vi "SPD.DT Meas DT_Grid.vi"(5 "Continue":refnum<vi>, 7 "Progress":refnum<vi>, 8 "Error In":errorcluster, 11 "SPD.Stand Ctrl in":T2={"spdDeviceSession"={"spdRef"=0, "connected"=FALSE, "spdName"="", "specification"={"diod case"=enum."default", "type"=enum."Unknown", "frequency"=enum."Unknown"}, "hidSPD.Controller"={"TSet"=0.0, "HV_bias"=0.0, "DDS_stb_code"=0}, "hidSPD.Sturtup Values"={"TSet"=0.0, "HV_bias"=0.0, "DDS_stb_code"=0}}, "DevBSession"={"DevBRef"="", "connected"=FALSE}, "FreqCSession"={"FreqCRef"="", "timeout"=0.0, "Gate"=0.0, "connected"=FALSE}, "8164BSession"={"Connection ID"=refnum, "Connected"=FALSE, "Info"="", "Slots Info"=[]}, "LeCroySession"={"LeCroySession"="", "connected"=FALSE}, "Events"={"DCRTest"=refnum, "Stop"=refnum}, "configFile"={"configFile ref"=refnum, "configFile path"=path "", "equipmentFile ref"=refnum}, "SPD.Meas Grid"={"DateTime"="", "DT"=[], "Insensitivity"=[], "Temprature"=[], "Stb_code"=[], "HV_Bias"=[]}, "SPD.Queues"={"state queue"=refnum}, "Console"=refnum} {"spdDeviceSession"."hidSPD.Sturtup Values"."HV_bias" format="%#_6p, V"; "spdDeviceSession"."hidSPD.Sturtup Values"."TSet" format="%#_6p, DegC"; "spdDeviceSession"."hidSPD.Controller"."HV_bias" format="%#_6p, V"; "spdDeviceSession"."hidSPD.Controller"."TSet" format="%#_6p, DegC"}) -> (0 "Error Out":errorcluster, 1 "pass":bool, 2 "Report":string, 3 "SPD.Stand Ctrl out":T2={"spdDeviceSession"={"spdRef"=0, "connected"=FALSE, "spdName"="", "specification"={"diod case"=enum."default", "type"=enum."Unknown", "frequency"=enum."Unknown"}, "hidSPD.Controller"={"TSet"=0.0, "HV_bias"=0.0, "DDS_stb_code"=0}, "hidSPD.Sturtup Values"={"TSet"=0.0, "HV_bias"=0.0, "DDS_stb_code"=0}}, "DevBSession"={"DevBRef"="", "connected"=FALSE}, "FreqCSession"={"FreqCRef"="", "timeout"=0.0, "Gate"=0.0, "connected"=FALSE}, "8164BSession"={"Connection ID"=refnum, "Connected"=FALSE, "Info"="", "Slots Info"=[]}, "LeCroySession"={"LeCroySession"="", "connected"=FALSE}, "Events"={"DCRTest"=refnum, "Stop"=refnum}, "configFile"={"configFile ref"=refnum, "configFile path"=path "", "equipmentFile ref"=refnum}, "SPD.Meas Grid"={"DateTime"="", "DT"=[], "Insensitivity"=[], "Temprature"=[], "Stb_code"=[], "HV_Bias"=[]}, "SPD.Queues"={"state queue"=refnum}, "Console"=refnum} {"spdDeviceSession"."hidSPD.Sturtup Values"."HV_bias" format="%#_6p, V"; "spdDeviceSession"."hidSPD.Sturtup Values"."TSet" format="%#_6p, DegC"; "spdDeviceSession"."hidSPD.Controller"."HV_bias" format="%#_6p, V"; "spdDeviceSession"."hidSPD.Controller"."TSet" format="%#_6p, DegC"})   [LabVIEW 2018]
uses:
  typedefs/SPD.Stand Ctrl.ctl
  Instruments/SPD HID Interface/hidSPDLibForLabView/LibVIs/hidSPD Controls/hidSPD Device Session.ctl
  Instruments/SPD HID Interface/hidSPDLibForLabView/LibVIs/hidSPD Controls/hidSPD.SPD specification.ctl
  Instruments/SPD HID Interface/hidSPDLibForLabView/LibVIs/hidSPD Controls/hidSPD SPD Diod Case.ctl
  Instruments/SPD HID Interface/hidSPDLibForLabView/LibVIs/hidSPD Controls/hidSPD SPD Type.ctl
  Instruments/SPD HID Interface/hidSPDLibForLabView/LibVIs/hidSPD Controls/hidSPD.STB Frequency.ctl
  Instruments/SPD HID Interface/hidSPDLibForLabView/LibVIs/hidSPD Controls/hidSPD Controller.ctl
  Instruments/KC705 DevBoard/typedefs/DevB.Session.ctl
  Instruments/KeySight 53230A/typedefs/FreqC.Session.ctl
  Instruments/KeySight 8164B/KeySight 8164B LAN InstrLib/typedefs/KeySight 8164B control.ctl
  Instruments/LeCroy SDA830/typedefs/LeCroy.Session.ctl
  typedefs/SPD.Events.ctl
  ConfigFile/SPD.Config File ctrl.ctl
  <vilib>/Utility/config.llb/Config Data RefNum.ctl
  typedefs/SPD.Meas Grid.ctl
  typedefs/SPD.Queues.ctl
  typedefs/SPD.Stand state.ctl
  typedefs/SPD.Common HW Setup ctr.ctl
  typedefs/SPD.QE Strobe_Phase Tune Limits.ctl
  <vilib>/Analysis/1siggen.llb/Ramp Pattern by Delta.vi
  <vilib>/Analysis/NI_AALBase.lvlib
  Instruments/KeySight 8164B/KeySight 8164B LAN InstrLib.lvlib
  <vilib>/Utility/config.llb/NI_LVConfig.lvlib
  Instruments/SPD HID Interface/hidSPDLibForLabView/hidSPDLibForLabView.lvlib
panel:
  out "XY Graph":T1(graph)
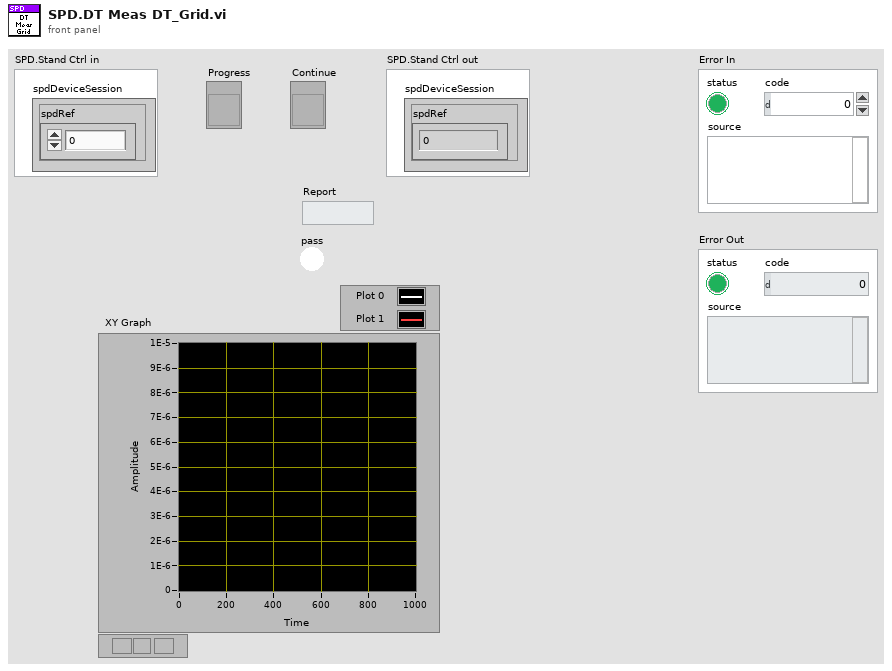
[diagram p1: front panel]
types:
  T1 = cluster{"result out":dbl[], "result out":dbl[]}[]
  T2 = typedef "SPD.Stand Ctrl.ctl" = cluster{"spdDeviceSession":T3, "DevBSession":T9, "FreqCSession":T10, "8164BSession":T11, "LeCroySession":T12, "Events":T13, "configFile":T14, "SPD.Meas Grid":T16, "SPD.Queues":T17, "Console":refnum<vi>}
  T3 = typedef "hidSPDLibForLabView.lvlib/hidSPD Device Session.ctl" = cluster{"spdRef":u64, "connected":bool, "spdName":string, "specification":T4, "hidSPD.Controller":T8, "hidSPD.Sturtup Values":T8}
  T4 = typedef "hidSPDLibForLabView.lvlib/hidSPD.SPD specification.ctl" = cluster{"diod case":T5, "type":T6, "frequency":T7}
  T5 = typedef "hidSPDLibForLabView.lvlib/hidSPD SPD Diod Case.ctl" = enum16{"Unknown", "default", "butterfly"}
  T6 = typedef "hidSPDLibForLabView.lvlib/hidSPD SPD Type.ctl" = enum16{"Unknown", "Free Run", "Gate"}
  T7 = typedef "hidSPDLibForLabView.lvlib/hidSPD.STB Frequency.ctl" = enum16{"Unknown", "312", "1250"}
  T8 = typedef "hidSPDLibForLabView.lvlib/hidSPD Controller.ctl" = cluster{"TSet":sgl, "HV_bias":sgl, "DDS_stb_code":u16}
  T9 = typedef "DevB.Session.ctl" = cluster{"DevBRef":refnum<visa-resource-name>, "connected":bool}
  T10 = typedef "FreqC.Session.ctl" = cluster{"FreqCRef":refnum<visa-resource-name>, "timeout":dbl, "Gate":dbl, "connected":bool}
  T11 = typedef "KeySight 8164B LAN InstrLib.lvlib/KeySight 8164B control.ctl" = cluster{"Connection ID":refnum<k5>, "Connected":bool, "Info":string, "Slots Info":string[]}
  T12 = typedef "LeCroy.Session.ctl" = cluster{"LeCroySession":refnum<visa-resource-name>, "connected":bool}
  T13 = typedef "SPD.Events.ctl" = cluster{"DCRTest":refnum<user-event>, "Stop":refnum<user-event>}
  T14 = typedef "SPD.Config File ctrl.ctl" = cluster{"configFile ref":T15, "configFile path":path, "equipmentFile ref":T15}
  T15 = typedef "NI_LVConfig.lvlib/Config Data RefNum.ctl" = refnum<k1>
  T16 = typedef "SPD.Meas Grid.ctl" = cluster{"DateTime":string, "DT":dbl[], "Insensitivity":dbl[], "Temprature":dbl[], "Stb_code":dbl[], "HV_Bias":dbl[][][][]}
  T17 = typedef "SPD.Queues.ctl" = cluster{"state queue":refnum<queue>}
  T18 = typedef "SPD.Common HW Setup ctr.ctl" = cluster{"FS":i32, "TS":i32, "Gate":dbl, "Att1 enable":bool, "Att3 enable":bool, "Att3 Att":dbl, "Scope setup file path":string, "Pset":dbl, "Set Pset":bool}
  T19 = typedef "SPD.DT&Insens Test Params.ctl" = cluster{"FS":i32, "TS":i32, "Att3":dbl, "Gate":dbl, "Num of Meas":i32, "ScopeRecallFile":string, "HistoSize":i32, "DT_min":u16, "DT_max":u16, "DT_step":u16, "Desired_DTs":dbl[], "Insens_bound":u16, "Insens_step":u16}
  T20 = typedef "SPD.QE Strobe_Phase Tune Limits.ctl" = cluster{"ph_start":i32, "ph_stop":i32, "ph_step":i32}
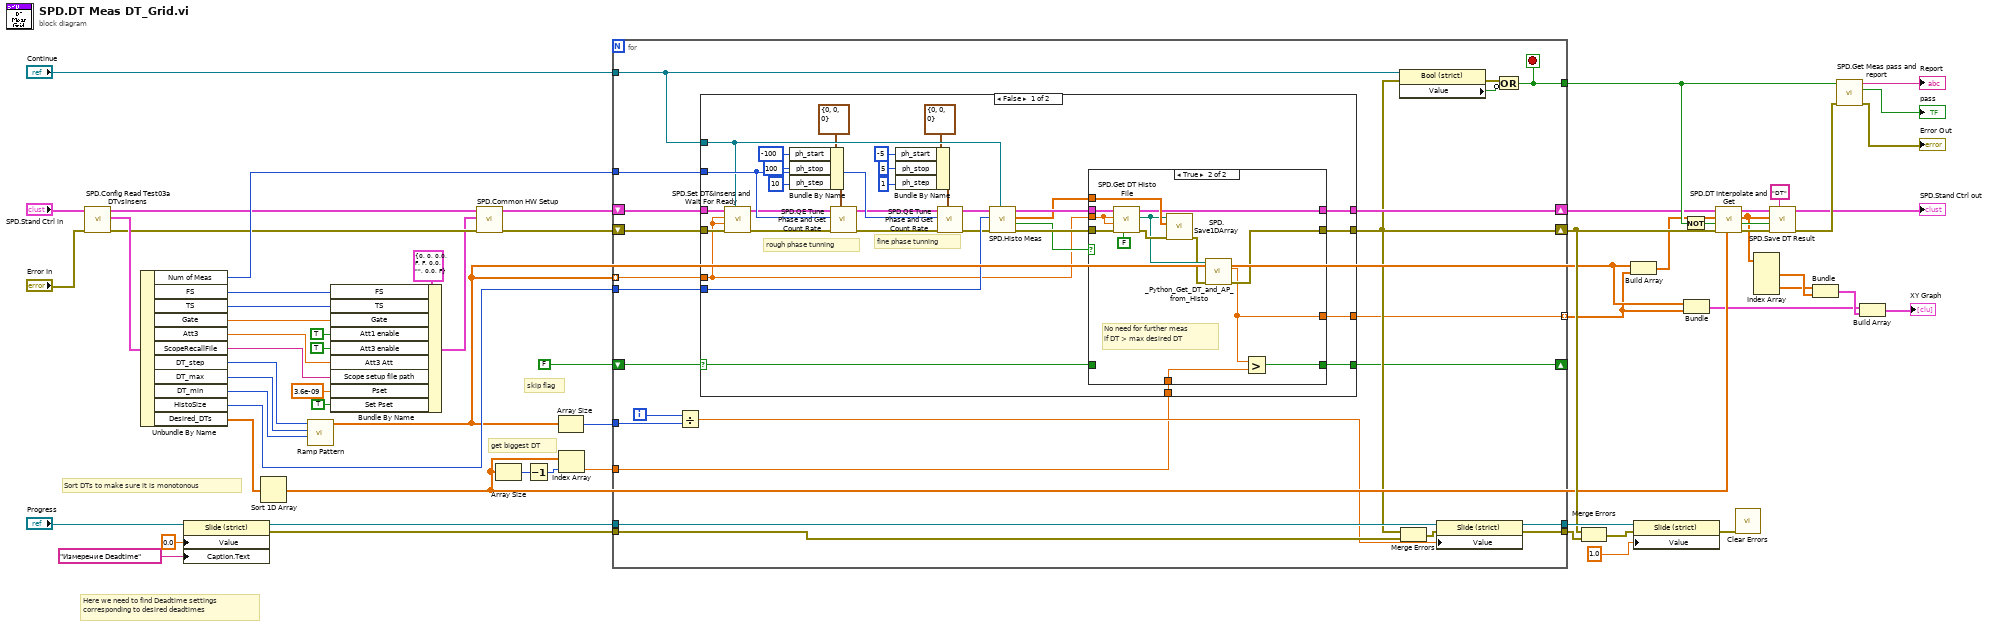
[diagram p0: block diagram]
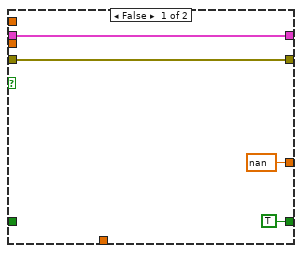
[diagram p2: hidden frame]
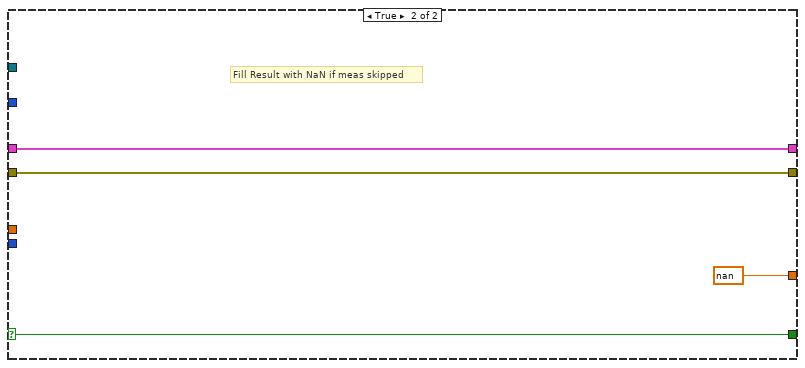
[diagram p3: hidden frame]
diagram:
  # "get biggest DT"
  # "Sort DTs to make sure it is monotonous"
  # "skip flag"
  # "Here we need to find Deadtime settings \ncorresponding to desired deadtimes"
  n1 = call "SPD.Config Read Test03a DTvsInsens.vi"("Error In"="Error In", "SPD.Stand Ctrl in"="SPD.Stand Ctrl in") -> ("Error Out"=w40:errorcluster, "DTvsInsens Params"=w41:T19, "SPD.Stand Ctrl out"=w43:T2)  [unwired: 7 in]
  n2 = Unbundle By Name(w41) -> ("Num of Meas"=w59:i32, "FS"=w48:i32, "TS"=w47:i32, "Gate"=w38:dbl, "Att3"=w37:dbl, "ScopeRecallFile"=w36:string, "DT_step"=w33:u16, "DT_max"=w32:u16, "DT_min"=w31:u16, "HistoSize"=w29:i32, "Desired_DTs"=w14:dbl[])
  n3 = property class="Slide (strict)"(reference="Progress", "Value"=0.0, "Caption.Text"="Измерение Deadtime") -> (reference out=w55:refnum<vi>, error out=w53:errorcluster)  [unwired: 1 in]
  n4 = Sort 1D Array(array=w14) -> (sorted array=w10:dbl[])
  n5 = call-poly <vilib>:"Ramp Pattern.vi"("start"=w31, "end"=w32, "delta"=w33) -> ("Ramp Pattern"=w8:dbl[])  [unwired: 6 in, 2 out]
  n6 = Bundle By Name(cluster=T18 {"FS"=0, "TS"=0, "Gate"=0.0, "Att1 enable"=FALSE, "Att3 enable"=FALSE, "Att3 Att"=0.0, "Scope setup file path"="", "Pset"=0.0, "Set Pset"=FALSE} ("common hw setup"), "FS"=w48, "TS"=w47, "Gate"=w38, "Att1 enable"=TRUE, "Att3 enable"=TRUE, "Att3 Att"=w37, "Scope setup file path"=w36, "Pset"=3.6e-09, "Set Pset"=TRUE) -> (w39:T18)
  n7 = call "SPD.Common HW Setup.vi"("error in (no error)"=w40, "common hw setup"=w39, "SPD.Stand Ctrl in in"=w43) -> ("error out"=w24:errorcluster, "SPD.Stand Ctrl out"=w23:T2)  [unwired: 7 in]
  n8 = Array Size(array=w10) -> (size(s)=w13:i32)
  n9 = Decrement(x=w13) -> (x-1=w12:i32)
  n10 = Array Size(array=w8) -> (size(s)=w30:i32)
  n11 = Index Array(array=w10, index=w12) -> (element=w11:dbl)
  n12 = for {
    shift-right: [w86] -> w26
    shift-left: w23 -> [w79]
    shift-right: [w70] -> w25
    shift-left: w24 -> [w78]
    tunnel: "Continue" -> [w77]
    tunnel: [w85] -> w28
    tunnel: w55 -> [w84]
    tunnel: [w83] -> w62
    tunnel: w59 -> [w82]
    tunnel: w53 -> [w81]
    tunnel: [w80] -> w51
    tunnel: w8 -> [w69] mode=indexing
    tunnel: w30 -> [w68]
    tunnel: w29 -> [w71]
    shift-right: [w66] -> _
    shift-left: FALSE -> [w67]
    tunnel: w11 -> [w65]
    tunnel: [w64] -> w7 mode=indexing
    i -> [w72]
    stop <- w85 stop-if-true
    n13 = Divide(x=w72, y=w68) -> (x/y=w74:dbl)
    n14 = case shown="False" w67 {
      selector: w67 -> [w90 w137]
      tunnel: [w118 w139] -> w86
      tunnel: w82 -> [w117 _]
      tunnel: w79 -> [w116 w139]
      tunnel: w78 -> [w114 w138]
      tunnel: w77 -> [w113 _]
      tunnel: w71 -> [w111 _]
      tunnel: [w92 w138] -> w70
      tunnel: w69 -> [w91 _]
      tunnel: [w87 nan] -> w64
      tunnel: [w89 w137] -> w66
      tunnel: w65 -> [w88 _]
      frame False {
        # "fine phase tunning"
        # "rough phase tunning"
        n15 = call "SPD.Set DT&Insens and Wait For Ready.vi"("Continue"=w113, "Error In"=w114, "insensitivity"=w91, "deadtime"=w91, "SPD.Stand Ctrl in"=w116) -> ("Error Out"=w112:errorcluster, "SPD.Stand Ctrl out"=w115:T2)  [unwired: 5 in]
        n16 = Bundle By Name(cluster=T20 {"ph_start"=0, "ph_stop"=0, "ph_step"=0} ("SPD.QE Strobe_Phase Tune Limits"), "ph_start"=-100, "ph_stop"=100, "ph_step"=10) -> (w95:T20)
        n17 = call "SPD.QE Tune Phase and Get Count Rate.vi"("SPD.QE Strobe_Phase Tune Limits"=w95, "Error In"=w112, "Num of FreqC Meas"=w117, "SPD.Stand Ctrl in"=w115) -> ("Error Out"=w100:errorcluster, "SPD.Stand Ctrl out"=w101:T2)  [unwired: 4 in, 2 out]
        n18 = Bundle By Name(cluster=T20 {"ph_start"=0, "ph_stop"=0, "ph_step"=0} ("SPD.QE Strobe_Phase Tune Limits"), "ph_start"=-5, "ph_stop"=5, "ph_step"=1) -> (w105:T20)
        n19 = call "SPD.QE Tune Phase and Get Count Rate.vi"("SPD.QE Strobe_Phase Tune Limits"=w105, "Error In"=w100, "Num of FreqC Meas"=w117, "SPD.Stand Ctrl in"=w101) -> ("Error Out"=w93:errorcluster, "SPD.Stand Ctrl out"=w94:T2)  [unwired: 4 in, 2 out]
        n20 = call "SPD.Histo Meas.vi"("Continue"=w113, "Error In"=w93, "Histo length"=w111, "SPD.Stand Ctrl in"=w94) -> ("Error Out"=w108:errorcluster, "pass"=w107:bool, "Histo"=w109:dbl[], "SPD.Stand Ctrl out"=w110:T2)  [unwired: 4 in]
        n21 = case shown="True" w107 {
          tunnel: [w122 w130] -> w118
          tunnel: [w121 w127] -> w92
          tunnel: w110 -> [w122 w135]
          tunnel: w109 -> [_ w132]
          tunnel: w108 -> [w121 w133]
          tunnel: w91 -> [_ w134]
          tunnel: [nan ("Dead Time") w123] -> w87
          tunnel: w90 -> [_ _]
          tunnel: [TRUE w126] -> w89
          tunnel: w88 -> [_ w124]
          frame False {
          }
          frame True {
            # "No need for further meas \nif DT > max desired DT"
            n22 = call "SPD.Get DT Histo File.vi"("DT folder"=FALSE, "Error In"=w133, "DT"=w134, "Insens"=w134, "SPD.Stand Ctrl in"=w135) -> ("Error Out"=w131:errorcluster, "DT Results path"=w129:path, "SPD.Stand Ctrl out"=w130:T2)  [unwired: 4 in]
            n23 = call "SPD.Save1DArray.vi"("Error In"=w131, "Array"=w132, "File Path"=w129) -> ("Error Out"=w128:errorcluster)  [unwired: 8 in]
            n24 = call "_Python_Get_DT_and_AP_from_Histo.vi"("error in (no error)"=w128, "Histo path"=w129) -> ("error out"=w127:errorcluster, "Dead Time"=w123:dbl)  [unwired: 7 in, 1 out]
            n25 = Greater?(x=w123, y=w124) -> (0:w126:bool)
          }
        }
      }
      frame True {
        # "Fill Result with NaN if meas skipped"
      }
    }
    n26 = property class="Bool (strict)"(reference=w77, error in=w70) -> (error out=w75:errorcluster, "Value"=w76:bool)  [unwired: 1 out]
    n27 = Merge Errors(w70, w81) -> (w73:errorcluster)
    n28 = property class="Slide (strict)"(reference=w84, error in=w73, "Value"=w74) -> (reference out=w83:refnum<vi>, error out=w80:errorcluster)
    n29 = Compound Arithmetic op=OR(w75, invert w76) -> (w85:bool)
  }
  n30 = Merge Errors(w25, w51) -> (w52:errorcluster)
  n31 = Build Array(w8, w7) -> (w9:dbl[][])
  n32 = property class="Slide (strict)"(reference=w62, error in=w52, "Value"=1.0) -> (error out=w60:errorcluster)  [unwired: 1 out]
  n33 = Not(x=w28) -> (.not. x?=w18:bool)
  n34 = Bundle("Ramp Pattern"=w8, w7) -> (w4:cluster{"Ramp Pattern":dbl[], dbl[]})  [unwired: 1 in]
  n35 = call "SPD.DT Interpolate and Get.vi"("desired DT"=w10, "Error In"=w25, "valid in"=w18, "Result"=w9, "SPD.Stand Ctrl in"=w26) -> ("Error Out"=w19:errorcluster, "valid out"=w17:bool, "result out"=w6:dbl[][], "SPD.Stand Ctrl out"=w20:T2)  [unwired: 3 in]
  n36 = call <vilib>:"Clear Errors.vi"("error in (no error)"=w60) -> ()  [unwired: 5 in, 2 out]
  n37 = Index Array(array=w6) -> (element #1=w2:dbl[], element #2=w1:dbl[])  [unwired: 4 in]
  n38 = call "SPD.Save DT Result.vi"("Name"="DT", "Error In"=w19, "write to file"=w17, "Result"=w6, "SPD.Stand Ctrl in"=w20) -> ("Error Out"=w16:errorcluster, "SPD.Stand Ctrl out"=→"SPD.Stand Ctrl out":T2)  [unwired: 5 in]
  n39 = Bundle("result out"=w1, "result out"=w2) -> (w5:cluster{"result out":dbl[], "result out":dbl[]})  [unwired: 1 in]
  n40 = call "SPD.Get Meas pass and report.vi"("error in (no error)"=w16, "error or stoped"=w28) -> ("error out"=→"Error Out":errorcluster, "pass"=→"pass":bool, "report"=→"Report":string)  [unwired: 7 in]
  n41 = Build Array(w4, w5) -> (→"XY Graph":T1)
